vi "Simple Cluster MsgPack Example.vi"() -> ()   [LabVIEW 2015, in "MsgPack.lvlib"]
uses:
  MsgPack.lvlib
  Simple Cluster.ctl
panel:
  in  "Key":string="Version"
  out "Key Found?":bool
  out "Received Packet":T1 {"Single" format="%#.19f"}
  out "Get Variant Attribute Error":errorcluster
  in  "Map to Cluster?(T)":bool=TRUE
  out "Decode Error":errorcluster
  out "Variant":variant
  in  "Cluster To Map? (T)":bool=TRUE
  in  "Flag":bool=TRUE
  in  "Compress? (T)":bool=TRUE
  out "MsgPack Data":string
  in  "Array Size":i32=20
  out "Packet":T1 {"Single" format="%#.19f"}
  # "This Example VI shows a way to send a simple Cluster over MsgPack.\n\nThe trick to decoding Clusters is the use of Variant Attributes.  During the decode phase an encoded MsgPack MAP is decoded as a true Key-Value look up table.  This can easily be  accessed using the \"Get Variant Attribute\" function.  This also allows for using default data if the sender didn't populate that particular key.\n\nFor this example to work without errors ensure the following parameters are TRUE:\n - Cluster To Map?\n - Map to Cluster?\n\n\"Cluster To Map?\" instructs the encoder to make a Key-Value pair (MsgPack MAP) of the input clusters data elements names/values.  The cluster must have unique names for every element.  See \"encodeCluster.vi\"\n  - True - Cluster is encoded as a MAP.\n  - False - Cluster is encoded as a heterogenous ARRAY.\n\n\"Map to Cluster?\" instructs the decoder to use Variant Attributes to build a Key-Value lookup table that is easy to parse.  See \"decodeMap.vi\"\n  - True - MsgPack MAP is decoded as a Key-Value table.  Keys must be unique STRINGS.   (More testing is needed to see if the KEY could be an integer, or some other data type.)\n  - False - MsgPack MAP is decoded as a 2D arrays, where the KEYS are in the first dimension, and the VALUES are in the second dimension. \n\n1 - Try setting different values for \"FLAG\" and \"Array Size\".\n2 - Toggle \"Compress?\"  to see the size difference in an array of integers\n3 - Toggle \"Cluster To Map?\" and \"Map To Cluster?\" to see how the MsgPack Data and resultant Variant are affected.\n4 - Try type in a new \"Key\" to see if it exists in the Variant.\n\n\nNote: Use Get Variant Attributes allows us to search the MsgPack packet for the matching key.  This allows the sending to not have to send all the keys, will the receiver can use default data for the \"missing\" keys.  This method is preferred because the MsgPack contract between the sender and receiver could be upgraded over time without breaking either side."
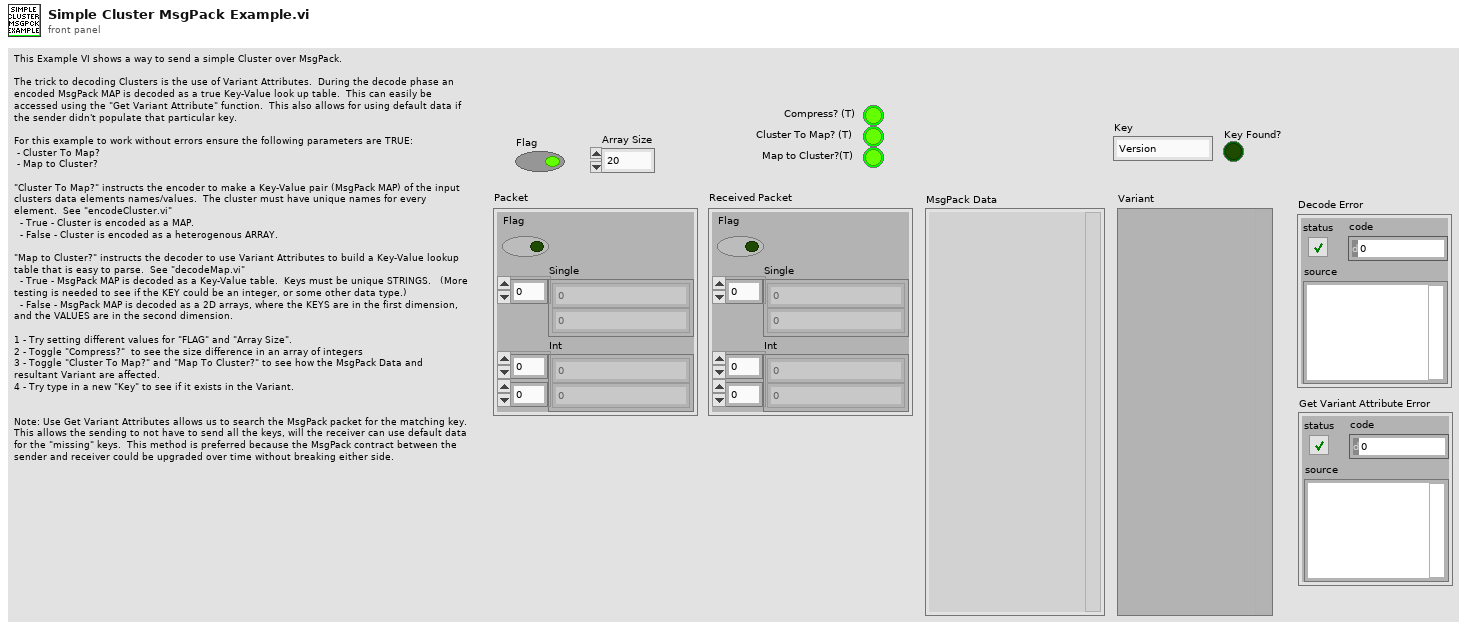
[diagram p1: front panel]
types:
  T1 = typedef "MsgPack.lvlib/Simple Cluster.ctl" = cluster{"Flag":bool, "Single":sgl[], "Int":i32[][]}
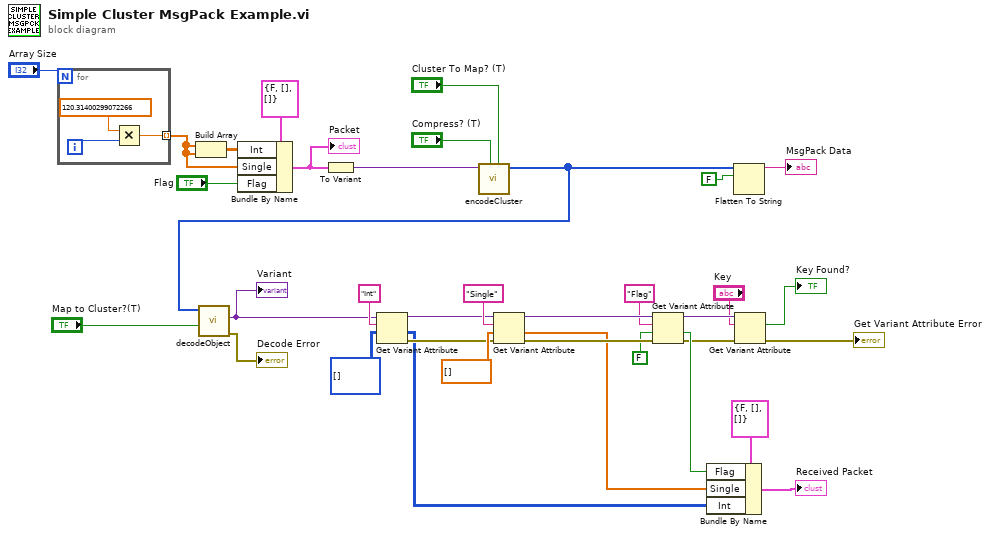
[diagram p0: block diagram]
diagram:
  n1 = for {
    N: "Array Size" -> [_]
    tunnel: [w37] -> w3 mode=indexing
    i -> [w38]
    n2 = Multiply(x=sgl 120.314, y=w38) -> (x*y=w37:sgl)
  }
  n3 = Build Array(w3, w3) -> (w2:sgl[][])
  n4 = Bundle By Name(cluster=T1 {"Flag"=FALSE, "Single"=[], "Int"=[]} ("Packet"), "Int"=w2, "Single"=w3, "Flag"="Flag") -> (w31:T1)
  "Packet" <- w31
  n5 = To Variant(anything=w31) -> (Variant=w30:variant)
  n6 = call "encodeCluster.vi"("Cluster To Map? [T]"="Cluster To Map? (T)", "Compress? (T)"="Compress? (T)", "Variant"=w30) -> ("MessagePack"=w11:u8[])  [unwired: 7 in, 1 out]
  n7 = call "decodeObject.vi"("Map to Cluster?(T)"="Map to Cluster?(T)", "ByteArray"=w11) -> ("error out"=→"Decode Error":errorcluster, "Variant"=w1:variant)  [unwired: 6 in, 2 out]
  "Variant" <- w1
  n8 = Get Variant Attribute(Variant=w1, name="Int", default value (empty Variant)=i32[][] []) -> (duplicate Variant=w14:variant, value=w12:i32[][], error out=w13:errorcluster)  [unwired: 1 in, 1 out]
  n9 = Get Variant Attribute(Variant=w14, name="Single", default value (empty Variant)=sgl[] [], error in=w13) -> (duplicate Variant=w23:variant, value=w9:sgl[], error out=w22:errorcluster)  [unwired: 1 out]
  n10 = Get Variant Attribute(Variant=w23, name="Flag", default value (empty Variant)=FALSE, error in=w22) -> (duplicate Variant=w6:variant, value=w10:bool, error out=w8:errorcluster)  [unwired: 1 out]
  n11 = Bundle By Name(cluster=T1 {"Flag"=FALSE, "Single"=[], "Int"=[]} ("Packet"), "Flag"=w10, "Single"=w9, "Int"=w12) -> (→"Received Packet":T1)
  n12 = Flatten To String(anything=w11, prepend array or string size? (T)=FALSE) -> (data string=→"MsgPack Data":string)  [unwired: 2 in, 2 out]
  n13 = Get Variant Attribute(Variant=w6, name="Key", error in=w8) -> (found=→"Key Found?":bool, error out=→"Get Variant Attribute Error":errorcluster)  [unwired: 1 in, 2 out]
